vi "dvp Vi Enum.vi"(9 "unSize":u32, 10 "friendlyName":string, 11 "index":u32) -> (2 "friendlyName out":string, 3 "function return":u32(ring))   [LabVIEW 2018, in "LabViewDVPCamera.lvlib"]
doc: "LabviewDvp2Api dvpStatus dvpViEnum(dvpUint32 index, char *friendlyName, dvpUint32 unSize);"
uses:
  LabViewDVPCamera.lvlib
  LabViewDVPCamera/LabViewDVPCamera.dll
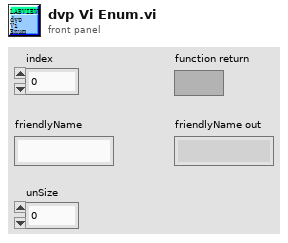
[diagram p1: front panel]
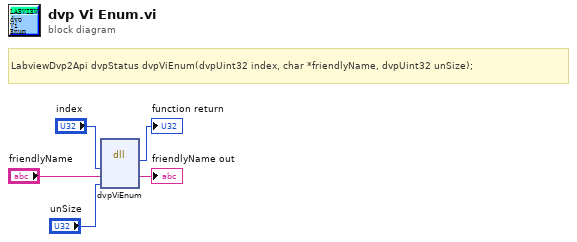
[diagram p0: block diagram]
diagram:
  # "LabviewDvp2Api dvpStatus dvpViEnum(dvpUint32 index, char *friendlyName, dvpUint32 unSize);"
  n1 = dll-call lib="C:/Program Files (x86)/DVP2 Labview cn 64/Sample/LabViewDVPCamera/LabViewDVPCamera.*" fn="dvpViEnum"("index"="index", "friendlyName"="friendlyName", "unSize"="unSize") -> (→"function return":u32, "friendlyName"=→"friendlyName out":string)  [unwired: 5 in, 2 out]
